vi "niRFUtil CAL Compute Calibration Loss.vi"(0 "Max Delta Frequency (Hz)":dbl=inf step=1000000.0 format="%^.6e", 1 "Max Delta Power Level (dBm)":dbl=inf step=10.0 format="%.1f", 2 "Table (frequency, power, pathloss)":T1 caption="Calibration Table [Hz, dBm, dB]" min=0 max=127 format="%.2p", 3 "Max Input Power (dBm)":dbl format="%.1f", 4 "Center Frequency (Hz)":dbl=1000000000.0 step=1000000.0 format="%^.6e") -> (5 "Max Frequency Delta Reached?":bool, 6 "Max Power Delta Reached?":bool, 7 "External Attenuation (dB)":dbl format="%.2f")   [LabVIEW 2015, in "niRFUtil.lvlib"]
uses:
  niRFUtil.lvlib
  Includes/niRFUtil INC Calibration Table.ctl
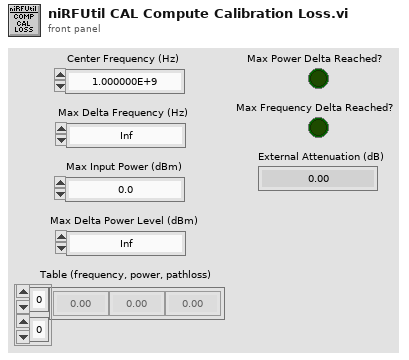
[diagram p1: front panel]
types:
  T1 = typedef "niRFUtil.lvlib/niRFUtil INC Calibration Table.ctl" = sgl[][]
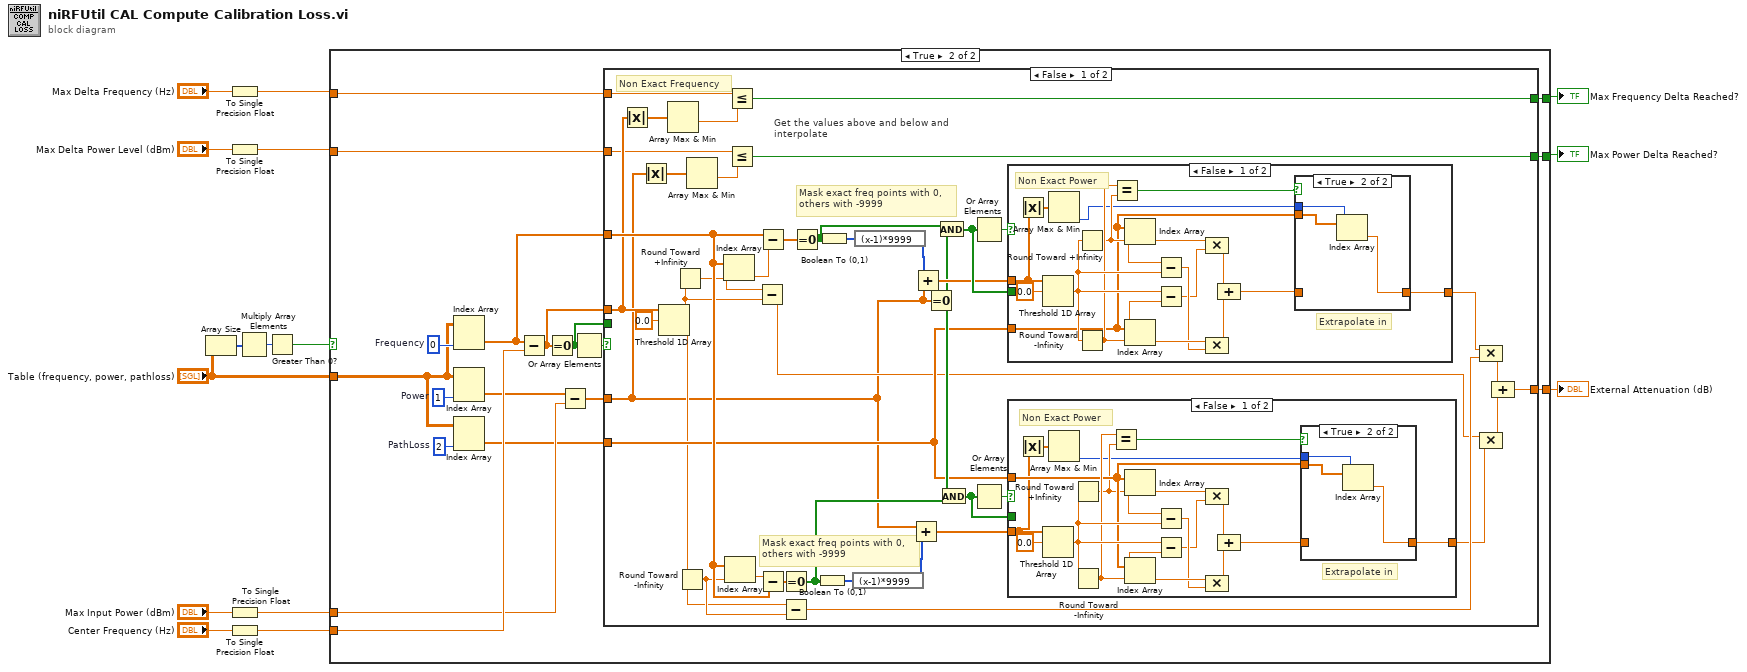
[diagram p0: block diagram]
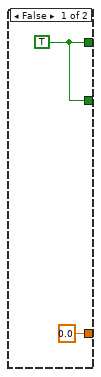
[diagram p2: hidden frame]
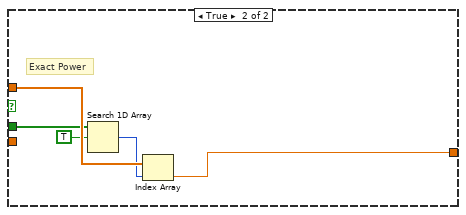
[diagram p4: hidden frame]
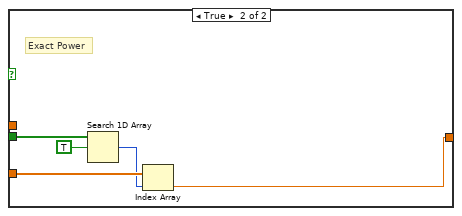
[diagram p6: hidden frame]
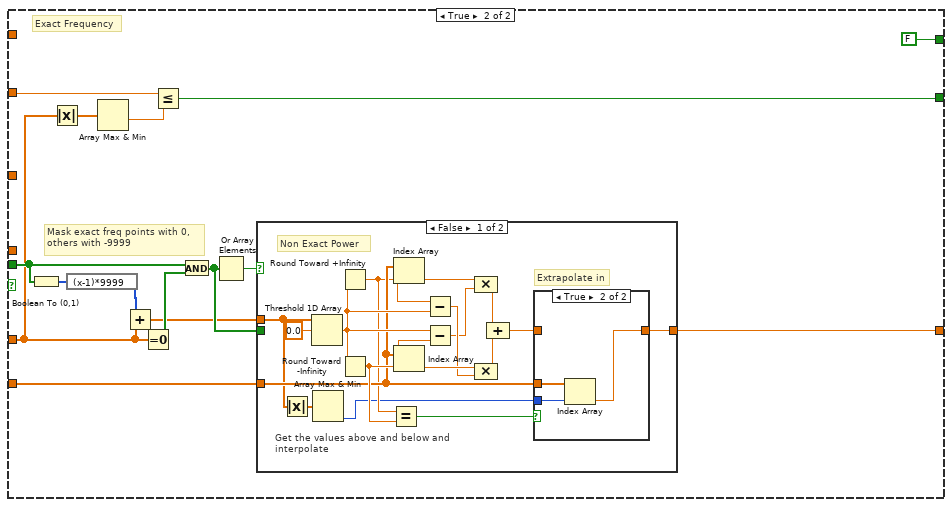
[diagram p7: hidden frame]
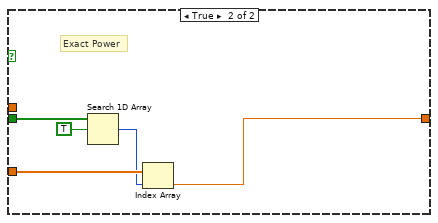
[diagram p9: hidden frame]
diagram:
  n1 = Array Size(array="Table (frequency, power, pathloss)") -> (size(s)=w7:i32[])
  n2 = To Single Precision Float(number="Max Delta Frequency (Hz)") -> (single precision float=w2:sgl)
  n3 = To Single Precision Float(number="Max Delta Power Level (dBm)") -> (single precision float=w1:sgl)
  n4 = To Single Precision Float(number="Max Input Power (dBm)") -> (single precision float=w4:sgl)
  n5 = To Single Precision Float(number="Center Frequency (Hz)") -> (single precision float=w3:sgl)
  n6 = Multiply Array Elements(1:w7) -> (0:w6:i32)
  n7 = Greater Than 0?(x=w6) -> (x > 0?=w5:bool)
  n8 = case shown="True" w5 {
    tunnel: [w17 w35] -> w15
    tunnel: [w17 w34] -> w14
    tunnel: w3 -> [_ w33]
    tunnel: w1 -> [_ w32]
    tunnel: w2 -> [_ w31]
    tunnel: w4 -> [_ w29]
    tunnel: [0.0 w27] -> w9
    tunnel: "Table (frequency, power, pathloss)" -> [_ w18]
    frame False {
      w17 = TRUE
    }
    frame True {
      w20 = 2  # PathLoss
      w19 = 0  # Frequency
      w21 = 1  # Power
      n9 = Index Array(array=w18, index (col)=w19) -> (element=w25:sgl[])  [unwired: 1 in]
      n10 = Index Array(array=w18, index (col)=w21) -> (element=w28:sgl[])  [unwired: 1 in]
      n11 = Index Array(array=w18, index (col)=w20) -> (element=w26:sgl[])  [unwired: 1 in]
      n12 = Subtract(x=w25, y=w33) -> (x-y=w24:sgl[])
      n13 = Equal To 0?(x=w24) -> (x = 0?=w23:bool[])
      n14 = Subtract(x=w28, y=w29) -> (x-y=w30:sgl[])
      n15 = Or Array Elements(Boolean array=w23) -> (logical OR=w22:bool)
      n16 = case shown="False" w22 {
        tunnel: w24 -> [w44 _]
        tunnel: w23 -> [_ w138]
        tunnel: w25 -> [w63 _]
        tunnel: w30 -> [w39 w130]
        tunnel: w26 -> [w57 w142]
        tunnel: [w47 w141] -> w27
        tunnel: w31 -> [w45 _]
        tunnel: w32 -> [w38 w131]
        tunnel: [w42 FALSE] -> w34
        tunnel: [w36 w129] -> w35
        frame False {
          # "Mask exact freq points with 0,\nothers with -9999"
          # "Mask exact freq points with 0,\nothers with -9999"
          # "Get the values above and below and\ninterpolate"
          # "Non Exact Frequency"
          n17 = Absolute Value(x=w44) -> (abs(x)=w43:sgl[])
          n18 = Absolute Value(x=w39) -> (abs(x)=w40:sgl[])
          n19 = Threshold 1D Array(2:0.0 ("threshold y"), 3:w44) -> (0:w48:sgl)  [unwired: 1 out]
          n20 = Array Max & Min(array=w43) -> (min value=w41:sgl)  [unwired: 3 out]
          n21 = Round Toward +Infinity(x=w48) -> (ceil(x): smallest int >= x=w49:sgl)
          n22 = Round Toward -Infinity(1:w48) -> (0:w50:sgl)
          n23 = Array Max & Min(array=w40) -> (min value=w37:sgl)  [unwired: 3 out]
          n24 = Index Array(array=w63, index=w49) -> (element=w46:sgl)
          n25 = Index Array(array=w63, index=w50) -> (element=w64:sgl)
          n26 = Less Or Equal?(x=w45, y=w41) -> (x <= y?=w42:bool)
          n27 = Less Or Equal?(x=w38, y=w37) -> (x <= y?=w36:bool)
          n28 = Subtract(x=w49, y=w48) -> (x-y=w51:sgl)
          n29 = Subtract(x=w63, y=w46) -> (x-y=w69:sgl[])
          n30 = Subtract(x=w64, y=w63) -> (x-y=w67:sgl[])
          n31 = Equal To 0?(x=w67) -> (x = 0?=w61:bool[])
          n32 = Subtract(x=w48, y=w50) -> (x-y=w56:sgl)
          n33 = Equal To 0?(x=w69) -> (x = 0?=w68:bool[])
          n34 = Boolean To (0,1)(Boolean=w61) -> (0, 1=w65:i16[])
          n35 = Boolean To (0,1)(Boolean=w68) -> (0, 1=w72:i16[])
          n36 = expression code="(x-1)*9999"(w65) -> (w66:i16[])
          n37 = expression code="(x-1)*9999"(w72) -> (w71:i16[])
          n38 = Add(x=w39, y=w66) -> (x+y=w58:sgl[])
          n39 = Add(x=w71, y=w39) -> (x+y=w70:sgl[])
          n40 = Equal To 0?(x=w39) -> (x = 0?=w62:bool[])
          n41 = And(x=w68, y=w62) -> (x .and. y?=w73:bool[])
          n42 = And(x=w62, y=w61) -> (x .and. y?=w59:bool[])
          n43 = Or Array Elements(Boolean array=w73) -> (logical OR=w74:bool)
          n44 = Or Array Elements(Boolean array=w59) -> (logical OR=w60:bool)
          n45 = case shown="False" w74 {
            tunnel: w57 -> [w107 w127]
            tunnel: [w105 w126] -> w53
            tunnel: w73 -> [_ w125]
            tunnel: w70 -> [w103 _]
            frame False {
              # "Extrapolate in"
              # "Non Exact Power"
              n46 = Absolute Value(x=w103) -> (abs(x)=w104:sgl[])
              n47 = Threshold 1D Array(2:0.0 ("threshold y"), 3:w103) -> (0:w115:sgl)  [unwired: 1 out]
              n48 = Array Max & Min(array=w104) -> (min index (indices)=w102:i32)  [unwired: 3 out]
              n49 = Round Toward +Infinity(x=w115) -> (ceil(x): smallest int >= x=w108:sgl)
              n50 = Round Toward -Infinity(1:w115) -> (0:w110:sgl)
              n51 = Equal?(x=w110, y=w108) -> (x = y?=w109:bool)
              n52 = Index Array(array=w107, index=w108) -> (element=w117:sgl)
              n53 = Index Array(array=w107, index=w110) -> (element=w116:sgl)
              n54 = Subtract(x=w108, y=w115) -> (x-y=w112:sgl)
              n55 = Subtract(x=w115, y=w110) -> (x-y=w111:sgl)
              n56 = Compound Arithmetic op=MULTIPLY(w117, w111) -> (w114:sgl)
              n57 = Compound Arithmetic op=MULTIPLY(w116, w112) -> (w113:sgl)
              n58 = Compound Arithmetic op=ADD(w114, w113) -> (w106:sgl)
              n59 = case shown="True" w109 {
                tunnel: w106 -> [w119 _]
                tunnel: [w119 w122] -> w105
                tunnel: w102 -> [_ w120]
                tunnel: w107 -> [_ w121]
                frame False {
                }
                frame True {
                  n60 = Index Array(array=w121, index=w120) -> (element=w122:sgl)
                }
              }
            }
            frame True {
              # "Exact Power"
              n61 = Search 1D Array(1D array=w125, element=TRUE) -> (index of element=w123:i32)  [unwired: 1 out]
              n62 = Index Array(array=w127, index=w123) -> (element=w126:sgl)
            }
          }
          n63 = case shown="False" w60 {
            tunnel: w57 -> [w80 w101]
            tunnel: [w83 w100] -> w52
            tunnel: w59 -> [_ w99]
            tunnel: w58 -> [w78 _]
            frame False {
              # "Extrapolate in"
              # "Non Exact Power"
              n64 = Absolute Value(x=w78) -> (abs(x)=w79:sgl[])
              n65 = Threshold 1D Array(2:0.0 ("threshold y"), 3:w78) -> (0:w89:sgl)  [unwired: 1 out]
              n66 = Array Max & Min(array=w79) -> (min index (indices)=w76:i32)  [unwired: 3 out]
              n67 = Round Toward +Infinity(x=w89) -> (ceil(x): smallest int >= x=w77:sgl)
              n68 = Round Toward -Infinity(1:w89) -> (0:w82:sgl)
              n69 = Equal?(x=w82, y=w77) -> (x = y?=w81:bool)
              n70 = Index Array(array=w80, index=w77) -> (element=w91:sgl)
              n71 = Index Array(array=w80, index=w82) -> (element=w90:sgl)
              n72 = Subtract(x=w77, y=w89) -> (x-y=w86:sgl)
              n73 = Subtract(x=w89, y=w82) -> (x-y=w85:sgl)
              n74 = Compound Arithmetic op=MULTIPLY(w91, w85) -> (w88:sgl)
              n75 = Compound Arithmetic op=MULTIPLY(w90, w86) -> (w87:sgl)
              n76 = Compound Arithmetic op=ADD(w88, w87) -> (w84:sgl)
              n77 = case shown="True" w81 {
                tunnel: w84 -> [w93 _]
                tunnel: [w93 w96] -> w83
                tunnel: w76 -> [_ w94]
                tunnel: w80 -> [_ w95]
                frame False {
                }
                frame True {
                  n78 = Index Array(array=w95, index=w94) -> (element=w96:sgl)
                }
              }
            }
            frame True {
              # "Exact Power"
              n79 = Search 1D Array(1D array=w99, element=TRUE) -> (index of element=w97:i32)  [unwired: 1 out]
              n80 = Index Array(array=w101, index=w97) -> (element=w100:sgl)
            }
          }
          n81 = Compound Arithmetic op=MULTIPLY(w53, w56) -> (w54:sgl)
          n82 = Compound Arithmetic op=MULTIPLY(w51, w52) -> (w55:sgl)
          n83 = Compound Arithmetic op=ADD(w54, w55) -> (w47:sgl)
        }
        frame True {
          # "Mask exact freq points with 0,\nothers with -9999"
          # "Exact Frequency"
          n84 = Boolean To (0,1)(Boolean=w138) -> (0, 1=w136:i16[])
          n85 = Absolute Value(x=w130) -> (abs(x)=w133:sgl[])
          n86 = expression code="(x-1)*9999"(w136) -> (w135:i16[])
          n87 = Array Max & Min(array=w133) -> (min value=w132:sgl)  [unwired: 3 out]
          n88 = Add(x=w135, y=w130) -> (x+y=w134:sgl[])
          n89 = Equal To 0?(x=w130) -> (x = 0?=w137:bool[])
          n90 = Less Or Equal?(x=w131, y=w132) -> (x <= y?=w129:bool)
          n91 = And(x=w138, y=w137) -> (x .and. y?=w139:bool[])
          n92 = Or Array Elements(Boolean array=w139) -> (logical OR=w140:bool)
          n93 = case shown="False" w140 {
            tunnel: w142 -> [w148 w168]
            tunnel: [w146 w167] -> w141
            tunnel: w139 -> [_ w166]
            tunnel: w134 -> [w145 _]
            frame False {
              # "Extrapolate in"
              # "Get the values above and below and\ninterpolate"
              # "Non Exact Power"
              n94 = Absolute Value(x=w145) -> (abs(x)=w144:sgl[])
              n95 = Threshold 1D Array(2:0.0 ("threshold y"), 3:w145) -> (0:w156:sgl)  [unwired: 1 out]
              n96 = Array Max & Min(array=w144) -> (min index (indices)=w143:i32)  [unwired: 3 out]
              n97 = Round Toward +Infinity(x=w156) -> (ceil(x): smallest int >= x=w147:sgl)
              n98 = Round Toward -Infinity(1:w156) -> (0:w151:sgl)
              n99 = Equal?(x=w147, y=w151) -> (x = y?=w150:bool)
              n100 = Index Array(array=w148, index=w147) -> (element=w158:sgl)
              n101 = Index Array(array=w148, index=w151) -> (element=w157:sgl)
              n102 = Subtract(x=w147, y=w156) -> (x-y=w153:sgl)
              n103 = Subtract(x=w156, y=w151) -> (x-y=w152:sgl)
              n104 = Compound Arithmetic op=MULTIPLY(w158, w152) -> (w155:sgl)
              n105 = Compound Arithmetic op=MULTIPLY(w157, w153) -> (w154:sgl)
              n106 = Compound Arithmetic op=ADD(w155, w154) -> (w149:sgl)
              n107 = case shown="True" w150 {
                tunnel: w149 -> [w160 _]
                tunnel: w148 -> [_ w163]
                tunnel: w143 -> [_ w162]
                tunnel: [w160 w161] -> w146
                frame False {
                }
                frame True {
                  n108 = Index Array(array=w163, index=w162) -> (element=w161:sgl)
                }
              }
            }
            frame True {
              # "Exact Power"
              n109 = Search 1D Array(1D array=w166, element=TRUE) -> (index of element=w164:i32)  [unwired: 1 out]
              n110 = Index Array(array=w168, index=w164) -> (element=w167:sgl)
            }
          }
        }
      }
    }
  }
  "Max Power Delta Reached?" <- w15
  "Max Frequency Delta Reached?" <- w14
  "External Attenuation (dB)" <- w9
